vi "IMMU - Simple Abs Val Filter.vi"(11 "Value In":dbl) -> (3 "Output":dbl)   [LabVIEW 2021]
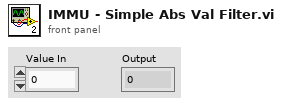
[diagram p1: front panel]
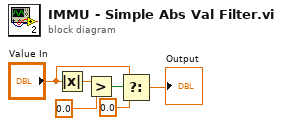
[diagram p0: block diagram]
diagram:
  n1 = Absolute Value(x="Value In") -> (abs(x)=w2:dbl)
  n2 = Greater?(x=w2, y=0.0) -> (0:w1:bool)
  n3 = Select(t="Value In", s=w1, f=0.0) -> (s? t:f=→"Output":dbl)
